vi "Import_Excel.vi"() -> ()   [LabVIEW 2019]
uses:
  <vilib>/Utility/NIReport.llb/Report Type.ctl
  <vilib>/addons/_office/excel.llb/Excel Get Data ([str]).vi
  <vilib>/Utility/NIReport.llb/NI_report.lvclass
  <vilib>/Utility/NIReport.llb/Excel/NI_Excel.lvclass
  <vilib>/addons/_office/NI_ReportGenerationToolkit.lvlib
  <vilib>/Utility/NIReport.llb/NI_ReportGenerationCore.lvlib
panel:
  out "data":string[][](array[string])
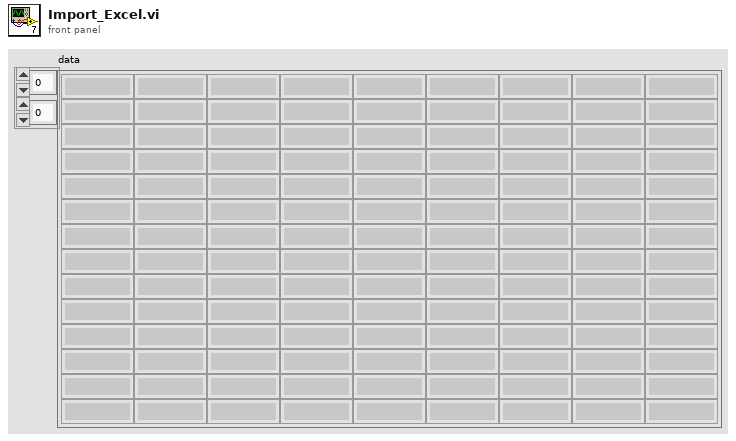
[diagram p1: front panel]
types:
  T1 = typedef "NI_ReportGenerationCore.lvlib/Report Type.ctl" = enum16{"HTML", "Word", "Excel"}
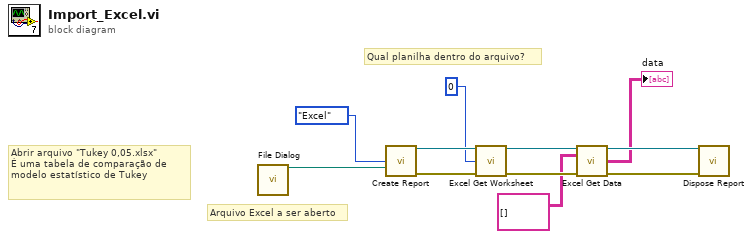
[diagram p0: block diagram]
diagram:
  # "Abrir arquivo \"Tukey 0,05.xlsx\"\nÉ uma tabela de comparação de modelo estatístico de Tukey"
  # "Qual planilha dentro do arquivo?"
  # "Arquivo Excel a ser aberto"
  n1 = call "File Dialog"() -> ("selected path"=w4:path)  [unwired: 12 in, 3 out]
  n2 = call <vilib>:"Create Report.vi"("report type"=Report_Type."Excel", "template (empty)"=w4) -> ("report out"=w11:refnum<class "NI_report.lvclass">, "error out"=w10:errorcluster)  [unwired: 12 in]
  n3 = call <vilib>:"Excel Get Worksheet.vi"("report in"=w11, "worksheet index (0)"=0, "error in (no error)"=w10) -> ("report out"=w9:refnum<class "NI_report.lvclass">, "error out"=w8:errorcluster)  [unwired: 11 in]
  n4 = call-poly <vilib>:"Excel Get Data.vi"("report in"=w9, "data type"=string[][] [] ("name (\"\")"), "error in (no error)"=w8) -> ("report out"=w7:refnum<class "NI_report.lvclass">, "data"=→"data":string[][], "error out"=w6:errorcluster)  [unwired: 10 in]
  n5 = call-dynamic "Dispose Report.vi"("report in"=w7, "error in (no error)"=w6) -> ()  [unwired: 13 in, 1 out]
